vi "Initialize.vi"(8 "error in (no error)":errorcluster, 9 "Reset (True)":bool=TRUE, 10 "ID Query (True)":bool=TRUE, 11 "VISA resource name":refnum<visa-resource-name>) -> (0 "error out":errorcluster, 3 "VISA resource name out":refnum<visa-resource-name>)   [LabVIEW 2014, in "Fluke 190 Series II.lvlib"]
doc: "Establishes communication with the instrument and optionally performs an instrument identification query and/or an instrument reset. It also places the instrument in a default state needed for other instrument driver operations. Therefore, call this VI before calling other instrument driver VIs for this instrument. Generally, you need to call the Initialize VI only once at the beginning of an application."
uses:
  Fluke 190 Series II.lvlib
panel:
  # "(c) 2013-2014 National Instruments.  ALL RIGHTS RESERVED."
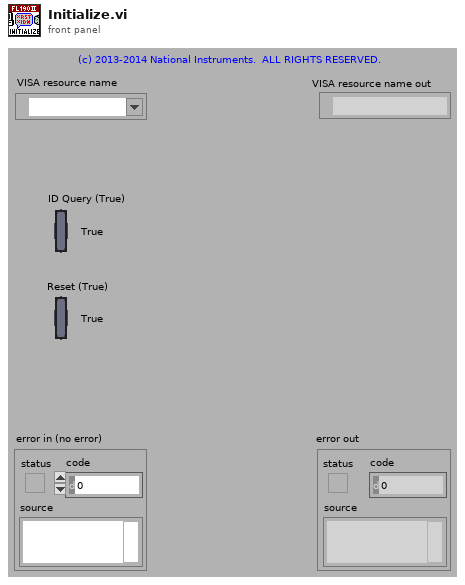
[diagram p1: front panel]
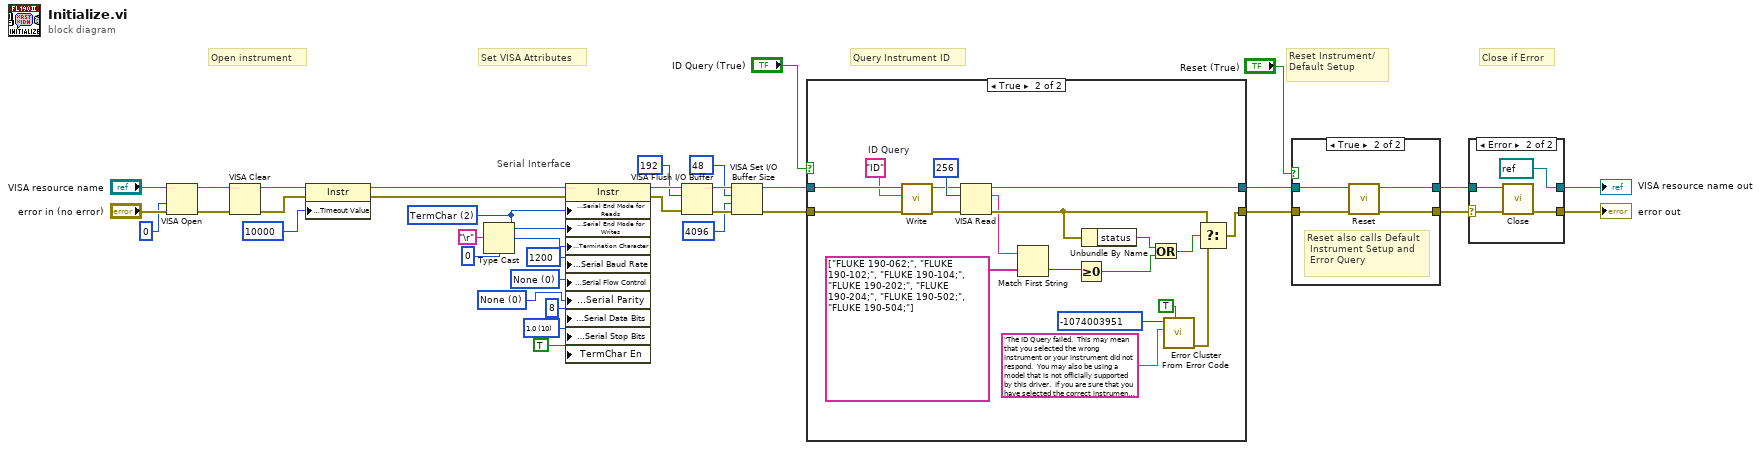
[diagram p0: block diagram]
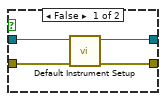
[diagram p3: hidden frame]
diagram:
  w3 = u16 0 items=["None", "XON/XOFF", "RTS/CTS", "XON/XOFF & RTS/CTS", "DTR/DSR", "XON/XOFF & DTR/DSR"] ("Serial Settings:Flow Control")
  w4 = u16 0 items=["None", "Odd", "Even", "Mark", "Space"] ("Serial Settings:Parity")
  w6 = u16 10 items=["1.0"=10, "1.5"=15, "2.0"=20] ("Serial Settings:Stop Bits")
  w9 = u16 2 items=["None", "LastBit", "TermChar"] ("Serial Settings:Serial End Mode for Reads")
  # "Serial Interface"
  # "Set VISA Attributes"
  # "Close if Error"
  # "Query Instrument ID"
  # "Reset Instrument/\nDefault Setup"
  # "Open instrument"
  n1 = VISA Open(access mode=u32 0, error in (no error)="error in (no error)", VISA resource name="VISA resource name") -> (VISA resource name=w25:refnum<visa-resource-name>, error out=w24:errorcluster)  [unwired: 2 out]
  n2 = VISA Clear(VISA resource name=w25, error in (no error)=w24) -> (VISA resource name out=w23:refnum<visa-resource-name>, error out=w22:errorcluster)
  n3 = property class="Instr"(reference=w23, error in=w22, "General Settings:Timeout Value"=u32 10000) -> (reference out=w28:refnum<visa-resource-name>, error out=w27:errorcluster)
  n4 = Type Cast(type=u8 0, x="\r") -> (*(type *) &x=w8:u8)
  n5 = property class="Instr"(reference=w28, error in=w27, "Serial Settings:Serial End Mode for Reads"=w9, "Serial Settings:Serial End Mode for Writes"=w9, "Message Based Settings:Termination Character"=w8, "Serial Settings:Serial Baud Rate"=u32 1200 ("Serial Settings:Baud Rate"), "Serial Settings:Serial Flow Control"=w3, "Serial Settings:Serial Parity"=w4, "Serial Settings:Serial Data Bits"=u16 8 ("Serial Settings:Data Bits"), "Serial Settings:Serial Stop Bits"=w6, "TermChar En"=TRUE ("Message Based Settings:Termination Character Enable")) -> (reference out=w14:refnum<visa-resource-name>, error out=w16:errorcluster)
  n6 = VISA Flush I/O Buffer(VISA resource name=w14, mask (16)=u16 192, error in (no error)=w16) -> (VISA resource name out=w17:refnum<visa-resource-name>, error out=w15:errorcluster)
  n7 = VISA Set I/O Buffer Size(VISA resource name=w17, mask (16)=u16 48, size (4096)=u32 4096 ("size (0)"), error in (no error)=w15) -> (VISA resource name out=w30:refnum<visa-resource-name>, error out=w29:errorcluster)
  n8 = case shown="True" "ID Query (True)" {
    tunnel: [w38 w58] -> w36
    tunnel: [w39 w57] -> w37
    tunnel: w30 -> [w39 w44]
    tunnel: w29 -> [w38 w43]
    frame False {
    }
    frame True {
      w40 = "ID"  # ID Query
      n9 = call "Write.vi"("error in (no error)"=w43, "Write Buffer"=w40, "VISA resource name"=w44) -> ("error out"=w41:errorcluster, "VISA resource name out"=w42:refnum<visa-resource-name>)  [unwired: 7 out]
      n10 = VISA Read(VISA resource name=w42, byte count=u32 256, error in (no error)=w41) -> (VISA resource name out=w57:refnum<visa-resource-name>, read buffer=w47:string, error out=w51:errorcluster)  [unwired: 1 out]
      n11 = Match First String(2:string[] ["FLUKE 190-062;", "FLUKE 190-102;", "FLUKE 190-104;", "FLUKE 190-202;", "FLUKE 190-204;", "FLUKE 190-502;", "FLUKE 190-504;"], 3:w47) -> (0:w45:i32)  [unwired: 1 out]
      n12 = Greater Or Equal To 0?(x=w45) -> (x >= 0?=w49:bool)
      n13 = Unbundle By Name(w51) -> ("status"=w50:bool)
      n14 = Or(x=w50, y=w49) -> (x .or. y?=w48:bool)
      n15 = call <vilib>:"Error Cluster From Error Code.vi"("show call chain? (False)"=TRUE, "error message (\"\")"="The ID Query failed.  This may mean that you selected the wrong instrument or your instrument did not respond.  You may also be using a model that is not officially supported by this driver.  If you are sure that you have selected the correct instrument and it is responding, try disabling the ID Query." ("Source (VI Name)"), "error code (0)"=-1074003951 ("Code")) -> ("error out"=w55:errorcluster)  [unwired: 1 in, 5 out]
      n16 = Select(t=w51, s=w48, f=w55) -> (s? t:f=w58:errorcluster)
    }
  }
  n17 = case shown="True" "Reset (True)" {
    tunnel: w36 -> [w61 w65]
    tunnel: [w59 w63] -> w18
    tunnel: w37 -> [w62 w66]
    tunnel: [w60 w64] -> w19
    frame False {
      n18 = call "Default Instrument Setup.vi"("error in (no error)"=w61, "VISA resource name"=w62) -> ("error out"=w59:errorcluster, "VISA resource name out"=w60:refnum<visa-resource-name>)  [unwired: 8 out]
    }
    frame True {
      # "Reset also calls Default\n Instrument Setup and\n Error Query"
      n19 = call "Reset.vi"("error in (no error)"=w65, "VISA resource name"=w66) -> ("error out"=w63:errorcluster, "VISA resource name out"=w64:refnum<visa-resource-name>)  [unwired: 8 out]
    }
  }
  n20 = case shown="Error" w18 {
    selector: w18 -> [w67 w70]
    tunnel: w19 -> [w68 w71]
    tunnel: [w68 refnum<visa-resource-name> refnum ("VISA resource name out")] -> w21
    tunnel: [w67 w72] -> w20
    frame No Error {
    }
    frame Error {
      n21 = call "Close.vi"("error in (no error)"=w70, "VISA resource name"=w71) -> ("error out"=w72:errorcluster)  [unwired: 9 out]
    }
  }
  "VISA resource name out" <- w21
  "error out" <- w20
